vi "interpolate.vi"(8 "error in (no error)":errorcluster, 10 "Counts In":dbl[](array[numeric]), 11 "Wavelengths In":dbl[](array[numeric])) -> (0 "error out":errorcluster, 2 "Wavelengths Out":dbl[](array[numeric]) format="%_6g", 3 "Counts Out":dbl[](array[numeric]) format="%_6g")   [LabVIEW 2013, in "AvaSpec.lvlib" / "AvaSpec Acquisition.lvlib"]
uses:
  AvaSpec Acquisition.lvlib
  <vilib>/Analysis/1siggen.llb/Ramp Pattern by Delta.vi
  <vilib>/gmath/NI_Gmath.lvlib
  <vilib>/Analysis/NI_AALBase.lvlib
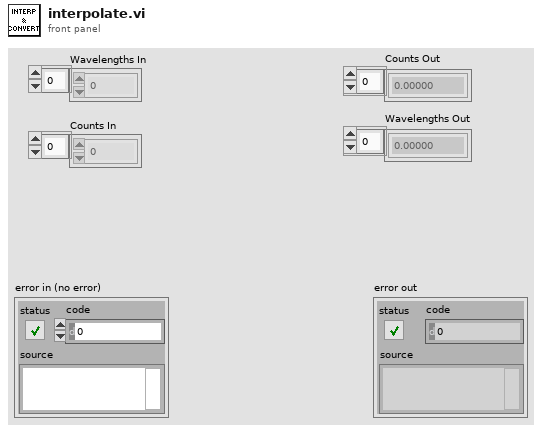
[diagram p1: front panel]
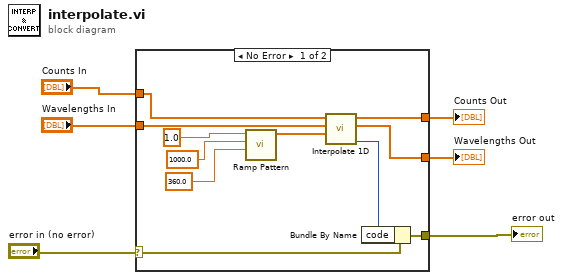
[diagram p0: block diagram]
diagram:
  n1 = case shown="No Error" "error in (no error)" {
    selector: "error in (no error)" -> [w9 w18]
    tunnel: [w13 _] -> w6
    tunnel: "Counts In" -> [w12 _]
    tunnel: "Wavelengths In" -> [w11 _]
    tunnel: [w10 _] -> w3
    tunnel: [w7 w18] -> w1
    frame No Error {
      n2 = call-poly <vilib>:"Ramp Pattern.vi"("start"=360.0, "end"=1000.0, "delta"=1.0) -> ("Ramp Pattern"=w17:dbl[])  [unwired: 6 in, 2 out]
      n3 = call <vilib>:"Interpolate 1D.vi"("xi"=w17, "X"=w11, "Y"=w12) -> ("error"=w8:i32, "xi used"=w10:dbl[], "yi"=w13:dbl[])  [unwired: 6 in]
      n4 = Bundle By Name(cluster=w9, "code"=w8) -> (w7:errorcluster)
    }
    frame Error {
    }
  }
  "Counts Out" <- w6
  "Wavelengths Out" <- w3
  "error out" <- w1
